vi "XBOX_Joystick_Name.vi"(10 "Buttons":bool[](array[boolean]), 11 "Axes":dbl[](array[numeric])) -> (2 "Named_Joystick":T2, 3 "Named_Buttons":T1)   [LabVIEW 2015]
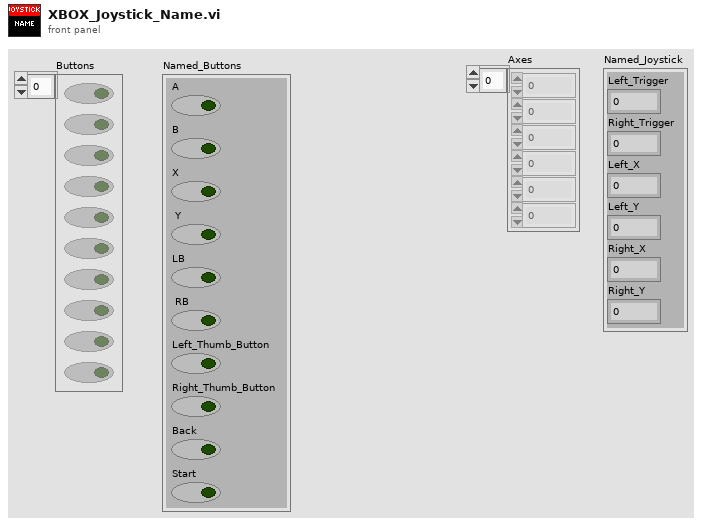
[diagram p1: front panel]
types:
  T1 = cluster{"A":bool, "B":bool, "X":bool, " Y":bool, "LB":bool, " RB":bool, "Left_Thumb_Button":bool, "Right_Thumb_Button":bool, "Back":bool, "Start":bool}
  T2 = cluster{"Left_Trigger":dbl, "Right_Trigger ":dbl, "Left_X":dbl, "Left_Y":dbl, "Right_X":dbl, "Right_Y":dbl}
  T3 = cluster{"Axes[0]":dbl, "Axes[1]":dbl, "Axes[2]":dbl, "Axes[3]":dbl, "Axes[4]":dbl, "Axes[5]":dbl}
  T4 = cluster{"Buttons[0]":bool, "Buttons[1]":bool, "Buttons[2]":bool, "Buttons[3]":bool, "Buttons[4]":bool, "Buttons[5]":bool, "Buttons[6]":bool, "Buttons[7]":bool, "Buttons[8]":bool, "Buttons[9]":bool}
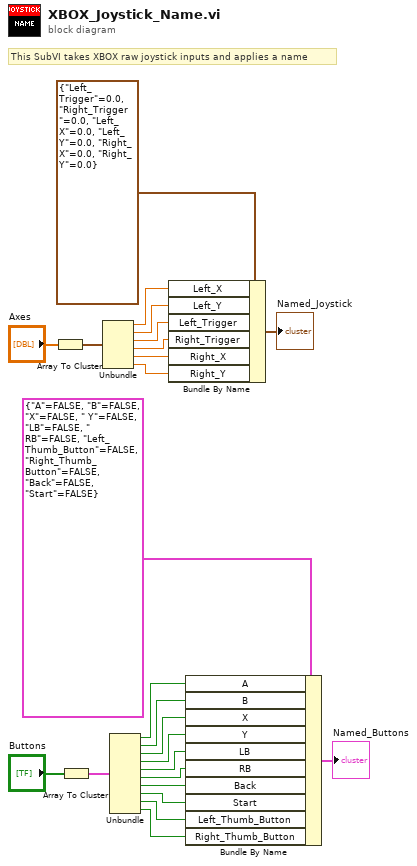
[diagram p0: block diagram]
diagram:
  # "This SubVI takes XBOX raw joystick inputs and applies a name"
  n1 = Array To Cluster(array="Axes") -> (cluster=w5:T3)
  n2 = Array To Cluster(array="Buttons") -> (cluster=w2:T4)
  n3 = Unbundle(w5) -> ("Axes[0]"=w18:dbl, "Axes[1]"=w19:dbl, "Axes[2]"=w20:dbl, "Axes[3]"=w21:dbl, "Axes[4]"=w22:dbl, "Axes[5]"=w23:dbl)
  n4 = Unbundle(w2) -> ("Buttons[0]"=w7:bool, "Buttons[1]"=w8:bool, "Buttons[2]"=w9:bool, "Buttons[3]"=w10:bool, "Buttons[4]"=w11:bool, "Buttons[5]"=w12:bool, "Buttons[6]"=w13:bool, "Buttons[7]"=w14:bool, "Buttons[8]"=w15:bool, "Buttons[9]"=w1:bool)
  n5 = Bundle By Name(cluster=T2 {"Left_Trigger"=0.0, "Right_Trigger "=0.0, "Left_X"=0.0, "Left_Y"=0.0, "Right_X"=0.0, "Right_Y"=0.0}, "Left_X"=w18, "Left_Y"=w19, "Left_Trigger"=w20, "Right_Trigger"=w21, "Right_X"=w22, "Right_Y"=w23) -> (→"Named_Joystick":T2)
  n6 = Bundle By Name(cluster=T1 {"A"=FALSE, "B"=FALSE, "X"=FALSE, " Y"=FALSE, "LB"=FALSE, " RB"=FALSE, "Left_Thumb_Button"=FALSE, "Right_Thumb_Button"=FALSE, "Back"=FALSE, "Start"=FALSE}, "A"=w7, "B"=w8, "X"=w9, "Y"=w10, "LB"=w11, "RB"=w12, "Back"=w13, "Start"=w14, "Left_Thumb_Button"=w15, "Right_Thumb_Button"=w1) -> (→"Named_Buttons":T1)
